vi "Tag Metadata Remove Group Zero Case.vi"(0 "Tags Array":string[][](array[string]), 7 "Boolean Refs Array":refnum<vi>[](array[refnum])) -> (4 "Updated Tag Array":string[][](array[string]), 15 "Current Tags":string[][](array[string]))   [LabVIEW 2020]
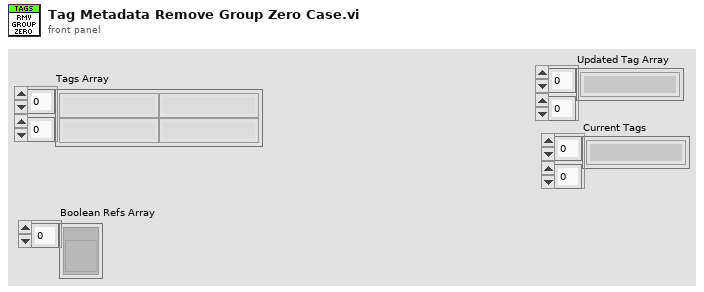
[diagram p1: front panel]
types:
  T1 = enum8{"Enabled", "Disabled", "Disabled and Grayed Out"}
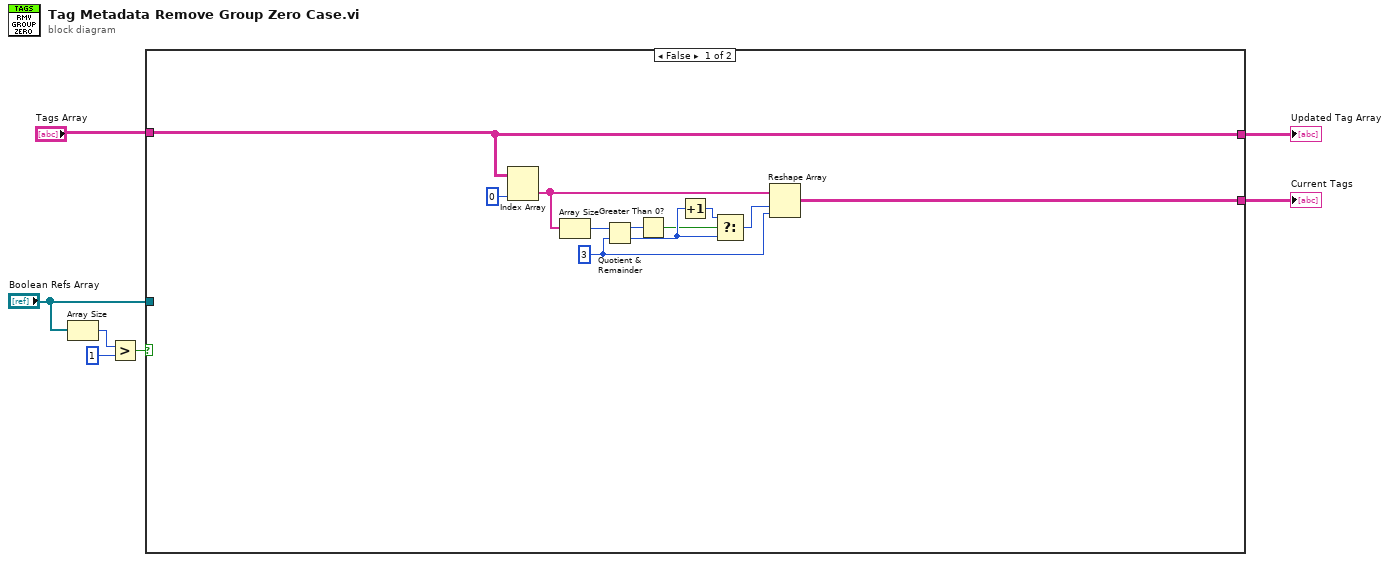
[diagram p0: block diagram]
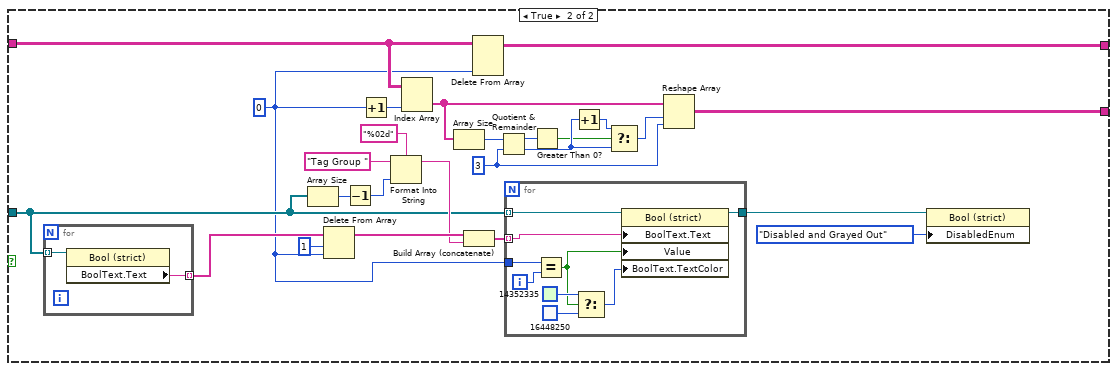
[diagram p2: hidden frame]
diagram:
  n1 = Array Size(array="Boolean Refs Array") -> (size(s)=w6:i32)
  n2 = Greater?(x=w6, y=1) -> (0:w4:bool)
  n3 = case shown="False" w4 {
    tunnel: "Boolean Refs Array" -> [_ w24]
    tunnel: "Tags Array" -> [w10 w22]
    tunnel: [w10 w21] -> w2
    tunnel: [w8 w20] -> w1
    frame False {
      w11 = 3 ("y")
      n4 = Index Array(array=w10, index (col)=0 ("disabled index (col)")) -> (element=w12:string[])  [unwired: 1 in]
      n5 = Array Size(array=w12) -> (size(s)=w13:i32)
      n6 = Quotient & Remainder(x=w13, y=w11) -> (x-y*floor(x/y)=w14:i32, floor(x/y)=w16:i32)
      n7 = Greater Than 0?(x=w14) -> (x > 0?=w15:bool)
      n8 = Increment(x=w16) -> (x+1=w17:i32)
      n9 = Select(t=w17, s=w15, f=w16) -> (s? t:f=w18:i32)
      n10 = Reshape Array(w12, w18, w11) -> (w8:string[][])
    }
    frame True {
      w19 = 0 ("Group Index")
      w26 = 3 ("y")
      n11 = for {
        tunnel: w24 -> [w45] mode=indexing
        tunnel: [w44] -> w23 mode=indexing
        n12 = property class="Bool (strict)"(reference=w45) -> ("BoolText.Text"=w44:string)  [unwired: 1 in, 2 out]
      }
      n13 = Array Size(array=w24) -> (size(s)=w39:i32)
      n14 = Delete From Array(array=w23, length=1, index=w19) -> (array with subset deleted=w42:string[])  [unwired: 1 out]
      n15 = Decrement(x=w39) -> (x-1=w36:i32)
      n16 = Increment(x=w19) -> (x+1=w25:i32)
      n17 = Format Into String(format string="%02d", initial string="Tag Group ", w36) -> (resulting string=w38:string)  [unwired: 1 in, 1 out]
      n18 = Index Array(array=w22, index (col)=w25) -> (element=w27:string[])  [unwired: 1 in]
      n19 = Array Size(array=w27) -> (size(s)=w28:i32)
      n20 = Build Array (concatenate)(w42, w38) -> (w37:string[])
      n21 = Delete From Array(array=w22, index (col)=w19) -> (array with subset deleted=w21:string[][])  [unwired: 2 in, 1 out]
      n22 = Quotient & Remainder(x=w28, y=w26) -> (x-y*floor(x/y)=w29:i32, floor(x/y)=w31:i32)
      n23 = for {
        tunnel: w24 -> [w54] mode=indexing
        tunnel: w37 -> [w51] mode=indexing
        tunnel: w19 -> [w53]
        tunnel: [w46] -> w34
        i -> [w52]
        n24 = Equal?(x=w53, y=w52) -> (x = y?=w48:bool)
        n25 = Select(t=u32 14352335 ("Color Box"), s=w48, f=u32 16448250) -> (s? t:f=w47:u32)
        n26 = property class="Bool (strict)"(reference=w54, "BoolText.Text"=w51, "Value"=w48, "BoolText.TextColor"=w47) -> (reference out=w46:refnum<vi>)  [unwired: 1 in, 1 out]
      }
      n27 = Greater Than 0?(x=w29) -> (x > 0?=w30:bool)
      n28 = Increment(x=w31) -> (x+1=w32:i32)
      n29 = Select(t=w32, s=w30, f=w31) -> (s? t:f=w33:i32)
      n30 = Reshape Array(w27, w33, w26) -> (w20:string[][])
      n31 = property class="Bool (strict)"(reference=w34, "DisabledEnum"=T1."Disabled and Grayed Out" ("Disabled")) -> ()  [unwired: 1 in, 2 out]
    }
  }
  "Updated Tag Array" <- w2
  "Current Tags" <- w1
